vi "Configure Measurement (Spectrum Monitor).vi"(0 "VISA resource name":refnum<visa-resource-name>, 5 "Reference Level (5 dBm)":i32=5 format="%^#_9g", 7 "Resolution Bandwidth (25E3 Hz)":dbl=25000.0 format="%^#_9g", 9 "Averaging Type (0: Log-Power Avg)":u16(ring) items=["Log-Power Avg", "Power Avg (RMS)"], 11 "error in (no error)":errorcluster) -> (4 "VISA resource name out":refnum<visa-resource-name>, 15 "error out":errorcluster)   [LabVIEW 2011, in "Agilent E5052X.lvlib"]
doc: "Configures the instrument to take Spectrum measurements.\n\n<b>Note: </b> \n\n\"Configure Measurement Characteristics(Spectrum)\" VI must be called before calling this VI."
uses:
  Agilent E5052X.lvlib
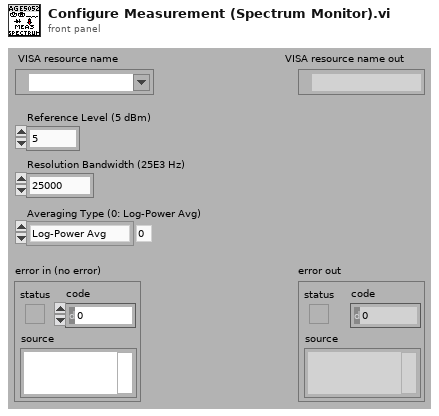
[diagram p1: front panel]
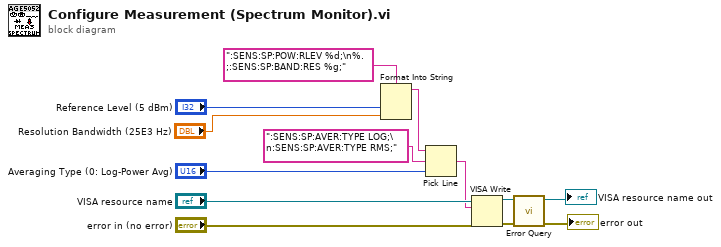
[diagram p0: block diagram]
diagram:
  n1 = Format Into String(format string=":SENS:SP:POW:RLEV %d;\n%.;:SENS:SP:BAND:RES %g;", "Reference Level (5 dBm)", "Resolution Bandwidth (25E3 Hz)") -> (resulting string=w3:string)  [unwired: 2 in, 1 out]
  n2 = Pick Line(string ("")=w3, multi-line string=":SENS:SP:AVER:TYPE LOG;\n:SENS:SP:AVER:TYPE RMS;", line index="Averaging Type (0: Log-Power Avg)") -> (output string=w1:string)
  n3 = VISA Write(VISA resource name="VISA resource name", write buffer=w1, error in (no error)="error in (no error)") -> (VISA resource name out=w8:refnum<visa-resource-name>, error out=w7:errorcluster)  [unwired: 1 out]
  n4 = call "Error Query.vi"("error in (no error)"=w7, "VISA resource name"=w8) -> ("error out"=→"error out":errorcluster, "VISA resource name out"=→"VISA resource name out":refnum<visa-resource-name>)  [unwired: 6 in, 2 out]
